vi "stop.vi"(8 "error in (no error)":errorcluster, 10 "Stop":bool, 11 "ICCameraAcquisitor in":refnum<class "ICCameraAcquisitor.lvclass">) -> (0 "error out":errorcluster, 2 "Stopped":bool=TRUE, 3 "ICCameraAcquisitor out":refnum<class "ICCameraAcquisitor.lvclass">)   [LabVIEW 2011, in "Hardware.lvlib" / "Channels.lvlib" / "ICCameraAcquisitor.lvclass"]
uses:
  ICCameraAcquisitor.lvclass
  ICCameraAcquisitor.lvclass/ICCameraAcquisitor.ctl
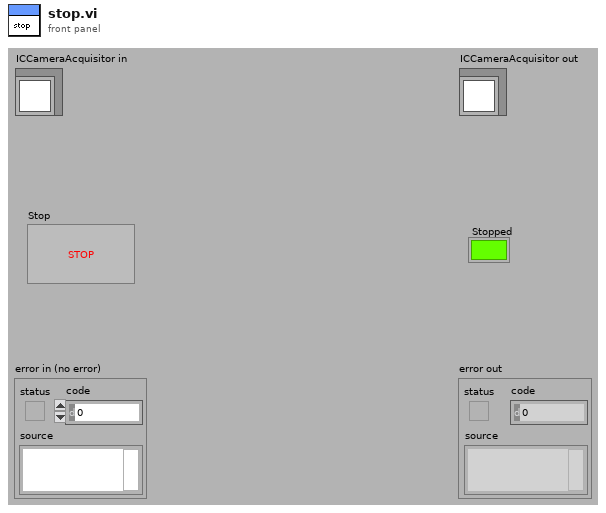
[diagram p1: front panel]
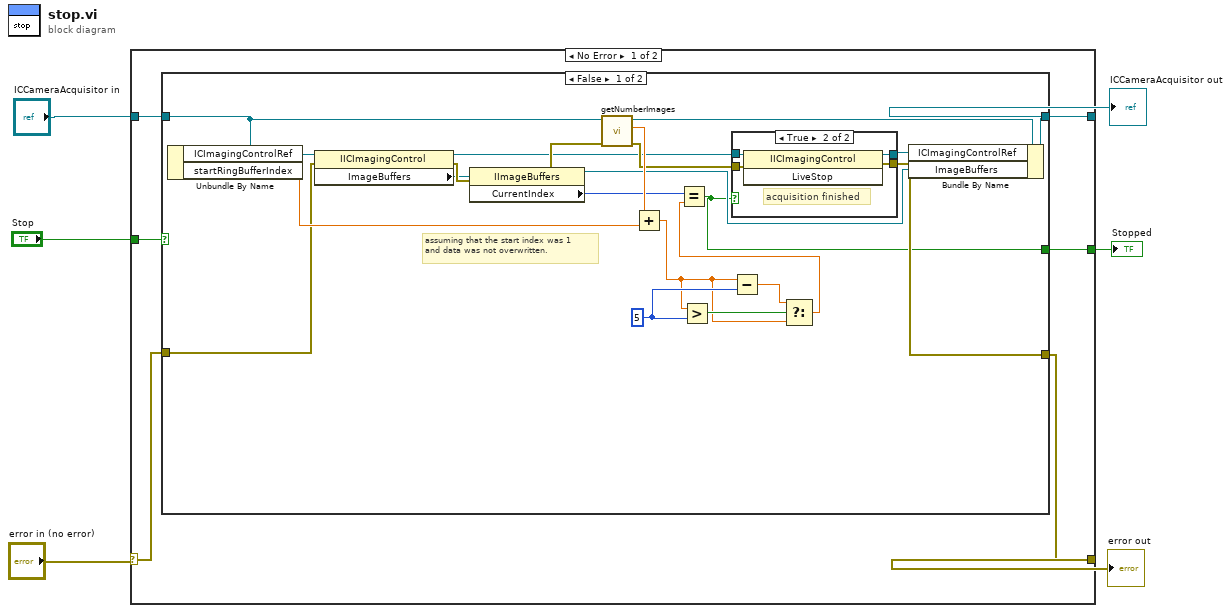
[diagram p0: block diagram]
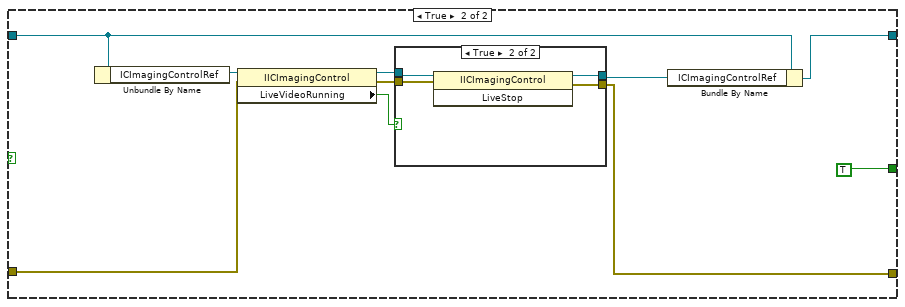
[diagram p3: hidden frame]
diagram:
  n1 = case shown="No Error" "error in (no error)" {
    selector: "error in (no error)" -> [w9 w57]
    tunnel: "ICCameraAcquisitor in" -> [w11 w58]
    tunnel: [w10 w58] -> w5
    tunnel: "Stop" -> [w12 _]
    tunnel: [w8 w57] -> w2
    tunnel: [w7 _] -> w1
    frame No Error {
      n2 = case shown="False" w12 {
        tunnel: w11 -> [w34 w46]
        tunnel: [w25 w45] -> w10
        tunnel: w9 -> [w22 w43]
        tunnel: [w26 w42] -> w8
        tunnel: [w13 TRUE] -> w7
        frame False {
          w19 = 5
          # "assuming that the start index was 1\nand data was not overwritten."
          n3 = Unbundle By Name(w34) -> ("ICImagingControlRef"=w24:refnum<k7>, "startRingBufferIndex"=w31:dbl)
          n4 = property class="IICImagingControl"(reference=w24, error in=w22) -> (reference out=w23:refnum<k7>, error out=w21:errorcluster, "ImageBuffers"=w20:refnum<k7>)
          n5 = property class="IImageBuffers"(reference=w20, error in=w21) -> (reference out=w27:refnum<k7>, error out=w33:errorcluster, "CurrentIndex"=w15:i32)
          n6 = call-dynamic "getNumberImages.vi"("error in (no error)"=w33, "CameraAcquisitor.lvclass in"=w34) -> ("error out"=w30:errorcluster, "Number of Images"=w32:dbl, "CameraAcquisitor.lvclass out"=w29:refnum<class "ICCameraAcquisitor.lvclass">)  [unwired: 7 in]
          n7 = Add(x=w32, y=w31) -> (x+y=w16:dbl)
          n8 = Greater?(x=w16, y=w19) -> (0:w17:bool)
          n9 = Subtract(x=w16, y=w19) -> (x-y=w18:dbl)
          n10 = Select(t=w18, s=w17, f=w16) -> (s? t:f=w14:dbl)
          n11 = Equal?(x=w15, y=w14) -> (x = y?=w13:bool)
          n12 = case shown="True" w13 {
            tunnel: w23 -> [w36 w40]
            tunnel: w30 -> [w35 w39]
            tunnel: [w36 w38] -> w28
            tunnel: [w35 w37] -> w26
            frame False {
              # "acquisition not finished"
            }
            frame True {
              # "acquisition finished"
              n13 = invoke class="IICImagingControl" method="LiveStop"(reference=w40, error in=w39) -> (reference out=w38:refnum<k7>, error out=w37:errorcluster)  [unwired: 1 in, 1 out]
            }
          }
          n14 = Bundle By Name(cluster=w29, "ICImagingControlRef"=w28, "ImageBuffers"=w27) -> (w25:refnum<class "ICCameraAcquisitor.lvclass">)
        }
        frame True {
          n15 = Unbundle By Name(w46) -> ("ICImagingControlRef"=w50:refnum<k7>)
          n16 = property class="IICImagingControl"(reference=w50, error in=w43) -> (reference out=w48:refnum<k7>, error out=w47:errorcluster, "LiveVideoRunning"=w49:bool)
          n17 = case shown="True" w49 {
            tunnel: w48 -> [w52 w56]
            tunnel: w47 -> [w51 w55]
            tunnel: [w52 w54] -> w44
            tunnel: [w51 w53] -> w42
            frame False {
            }
            frame True {
              n18 = invoke class="IICImagingControl" method="LiveStop"(reference=w56, error in=w55) -> (reference out=w54:refnum<k7>, error out=w53:errorcluster)  [unwired: 1 in, 1 out]
            }
          }
          n19 = Bundle By Name(cluster=w46, "ICImagingControlRef"=w44) -> (w45:refnum<class "ICCameraAcquisitor.lvclass">)
        }
      }
    }
    frame Error {
    }
  }
  "error out" <- w2
  "ICCameraAcquisitor out" <- w5
  "Stopped" <- w1
